vi "GetTerms4 1.vi"(0 "XRef":T11, 1 "State In":T10) -> (14 "Terms":T2, 15 "Fatal Error Out":T1)   [LabVIEW 2012, in "VireoFunctionNode.xnode"]
uses:
  VireoFunctionNode.xnode
  <vilib>/XNodeSupport/XNodeXNodeRef.ctl
  State 1.ctl
  <vilib>/XNodeSupport/XNodeTerm4Array.ctl
  <vilib>/XNodeSupport/XNodeTerm4.ctl
  <vilib>/XNodeSupport/XNodeString.ctl
  <vilib>/XNodeSupport/XNodeVariant.ctl
  <vilib>/XNodeSupport/XNodeRect32.ctl
  <vilib>/XNodeSupport/XNodeInt.ctl
  <vilib>/XNodeSupport/XNodeBool.ctl
  <vilib>/XNodeSupport/XNodeTermDirection.ctl
  <vilib>/XNodeSupport/XNodeErrorCluster.ctl
  <vilib>/XNodeSupport/NI_XNodeSupport.lvlib
  <vilib>/Utility/VariantDataType/VariantType.lvlib
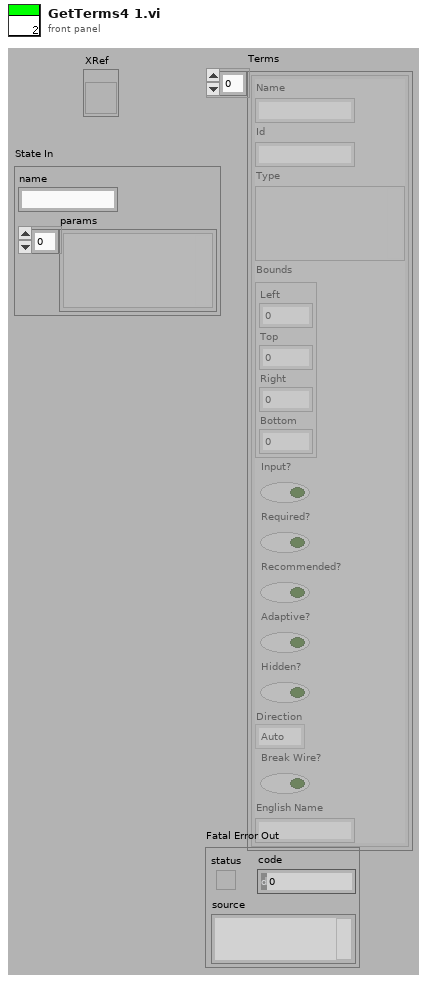
[diagram p1: front panel]
types:
  T1 = typedef "NI_XNodeSupport.lvlib/XNodeErrorCluster.ctl" = errorcluster
  T2 = typedef "NI_XNodeSupport.lvlib/XNodeTerm4Array.ctl" = T3[]
  T3 = typedef "NI_XNodeSupport.lvlib/XNodeTerm4.ctl" = cluster{"Name":T4, "Id":T4, "Type":T5, "Bounds":T6, "Input?":T8, "Required?":T8, "Recommended?":T8, "Adaptive?":T8, "Hidden?":T8, "Direction":T9, "Break Wire?":T8, "English Name":T4}
  T4 = typedef "NI_XNodeSupport.lvlib/XNodeString.ctl" = string
  T5 = typedef "NI_XNodeSupport.lvlib/XNodeVariant.ctl" = variant
  T6 = typedef "NI_XNodeSupport.lvlib/XNodeRect32.ctl" = cluster{"Left":T7, "Top":T7, "Right":T7, "Bottom":T7}
  T7 = typedef "NI_XNodeSupport.lvlib/XNodeInt.ctl" = i32
  T8 = typedef "NI_XNodeSupport.lvlib/XNodeBool.ctl" = bool
  T9 = typedef "NI_XNodeSupport.lvlib/XNodeTermDirection.ctl" = enum32{"Auto", "Up", "Down", "Left", "Right", "Center"}
  T10 = typedef "VireoFunctionNode.xnode/State 1.ctl" = cluster{"name":string, "params":variant[]}
  T11 = typedef "NI_XNodeSupport.lvlib/XNodeXNodeRef.ctl" = refnum<vi>
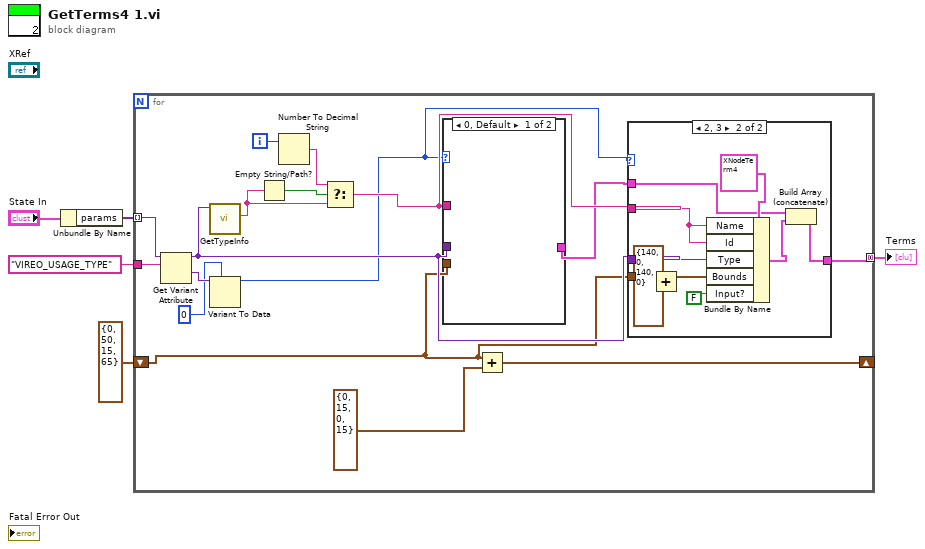
[diagram p0: block diagram]
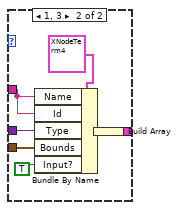
[diagram p3: hidden frame]
diagram:
  n1 = Unbundle By Name("State In") -> ("params"=w4:variant[])
  n2 = for {
    tunnel: w4 -> [w15] mode=indexing
    tunnel: [w6] -> w3 mode=concatenating
    shift-right: [w20] -> _
    shift-left: T6 {"Left"=0, "Top"=50, "Right"=15, "Bottom"=65} ("Bounds") -> [w9]
    tunnel: "VIREO_USAGE_TYPE" ("name") -> [w14]
    i -> [w19]
    n3 = Get Variant Attribute(Variant=w15, name=w14) -> (duplicate Variant=w10:variant, value=w13:variant)  [unwired: 2 in, 2 out]
    n4 = call <vilib>:"GetTypeInfo.vi"("Variant"=w10) -> ("Name"=w16:string)  [unwired: 6 in, 4 out]
    n5 = Variant To Data(type=0, Variant=w13) -> (data=w7:i32)  [unwired: 1 in, 1 out]
    n6 = Empty String/Path?(string/path=w16) -> (empty?=w18:bool)
    n7 = Number To Decimal String(number=w19) -> (decimal integer string=w17:string)  [unwired: 1 in]
    n8 = Select(t=w17, s=w18, f=w16) -> (s? t:f=w11:string)
    n9 = case shown="0, Default" w7 {
      tunnel: [_ w33] -> w8
      tunnel: w9 -> [_ w36]
      tunnel: w11 -> [_ w35]
      tunnel: w10 -> [_ w34]
      frame 0, Default {
      }
      frame 1, 3 {
        n10 = Bundle By Name(cluster=T3 {"Name"="", "Id"="", "Type"=variant, "Bounds"={"Left"=0, "Top"=0, "Right"=0, "Bottom"=0}, "Input?"=FALSE, "Required?"=FALSE, "Recommended?"=FALSE, "Adaptive?"=FALSE, "Hidden?"=FALSE, "Direction"=enum."Auto", "Break Wire?"=FALSE, "English Name"=""} ("Term 4"), "Name"=w35, "Id"=w35, "Type"=w34, "Bounds"=w36, "Input?"=T8 TRUE) -> (w38:T3)
        n11 = Build Array(w38) -> (w33:T3[])
      }
    }
    n12 = Add(x=w9, y=T6 {"Left"=0, "Top"=15, "Right"=0, "Bottom"=15}) -> (x+y=w20:T6)
    n13 = case shown="2, 3" w7 {
      tunnel: [w22 w23] -> w6
      tunnel: w9 -> [_ w30]
      tunnel: w11 -> [_ w29]
      tunnel: w10 -> [_ w28]
      tunnel: w8 -> [w22 w25]
      frame 0, Default {
      }
      frame 2, 3 {
        n14 = Add(x=w30, y=T6 {"Left"=140, "Top"=0, "Right"=140, "Bottom"=0}) -> (x+y=w27:T6)
        n15 = Bundle By Name(cluster=T3 {"Name"="", "Id"="", "Type"=variant, "Bounds"={"Left"=0, "Top"=0, "Right"=0, "Bottom"=0}, "Input?"=FALSE, "Required?"=FALSE, "Recommended?"=FALSE, "Adaptive?"=FALSE, "Hidden?"=FALSE, "Direction"=enum."Auto", "Break Wire?"=FALSE, "English Name"=""} ("Term 4"), "Name"=w29, "Id"=w29, "Type"=w28, "Bounds"=w27, "Input?"=T8 FALSE) -> (w24:T3)
        n16 = Build Array (concatenate)(w25, w24) -> (w23:T3[])
      }
    }
  }
  "Terms" <- w3
